vi "Set Connection Info.vi"(8 "error in (no error)":errorcluster, 10 "connection info":T1={"host"="3.128.20.209", "port"="5432", "dbname"="levylab", "user"="reader", "password"=""}, 11 "Data.PG in":refnum<class "Data.PG.lvclass">) -> (0 "error out":errorcluster, 3 "Data.PG out":refnum<class "Data.PG.lvclass">)   [LabVIEW 2020, in "Data.PG.lvclass"]
uses:
  Data.PG.lvclass
  Data.PG.lvclass/Data.PG.ctl
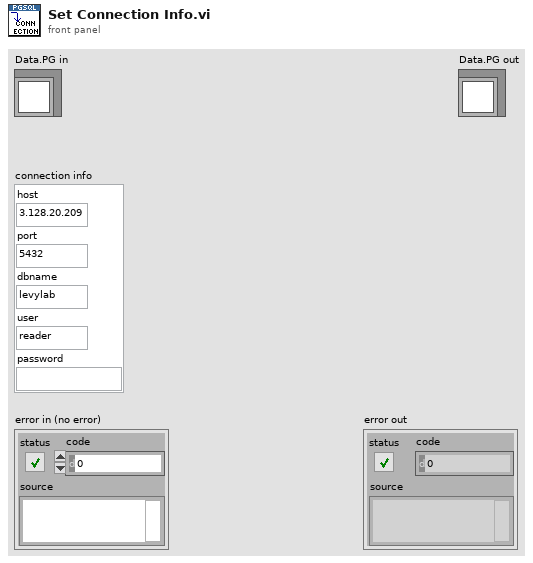
[diagram p1: front panel]
types:
  T1 = cluster{"host":string, "port":string, "dbname":string, "user":string, "password":string}
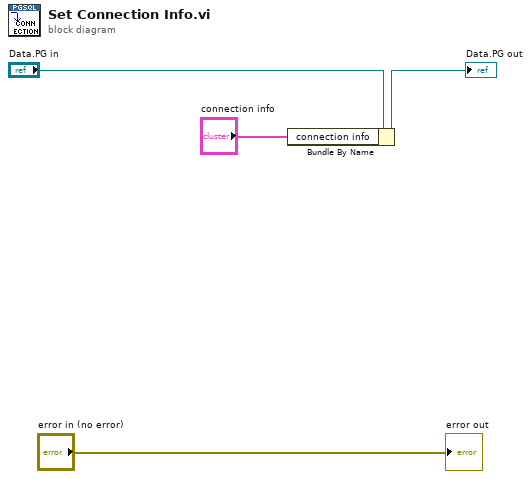
[diagram p0: block diagram]
diagram:
  n1 = Bundle By Name(cluster="Data.PG in", "connection info"="connection info") -> (→"Data.PG out":refnum<class "Data.PG.lvclass">)
  "error out" <- "error in (no error)"
